vi "Convert Celcius to Fahrenheit.vi"(1 "Tc":dbl) -> (0 "Tf":dbl)   [LabVIEW 2017]
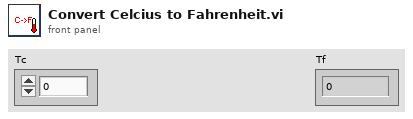
[diagram p1: front panel]
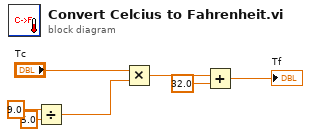
[diagram p0: block diagram]
diagram:
  n1 = Divide(x=9.0, y=5.0) -> (x/y=w4:dbl)
  n2 = Multiply(x="Tc", y=w4) -> (x*y=w3:dbl)
  n3 = Add(x=w3, y=32.0) -> (x+y=→"Tf":dbl)
